vi "Configure PA UTSIGNAL.vi"(8 "error in (no error)":errorcluster, 9 "OFF/ON":u8 max=1 step=1, 10 "Step":T1=1 min=1 max=99 step=1, 11 "VISA resource in":refnum<visa-resource-name>) -> (0 "error out":errorcluster, 3 "VISA resource out":refnum<visa-resource-name>)   [LabVIEW 2025, in "Chroma 19052.lvlib"]
uses:
  <instrlib>/Chroma 19052/Chroma 19052.lvlib
  <instrlib>/Chroma 19052/Public/Utility/Type Def/steps--numeric.ctl
panel:
  # "Set UT SIGNAL on/off"
  # "0 = OFF\n1 = ON"
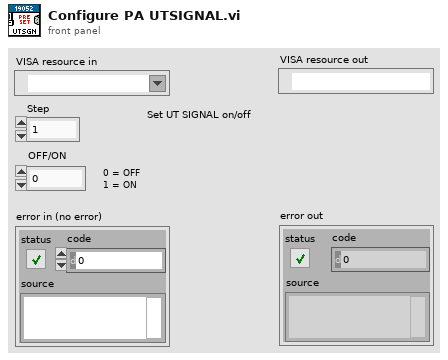
[diagram p1: front panel]
types:
  T1 = typedef "Chroma 19052.lvlib/steps--numeric.ctl" = u8
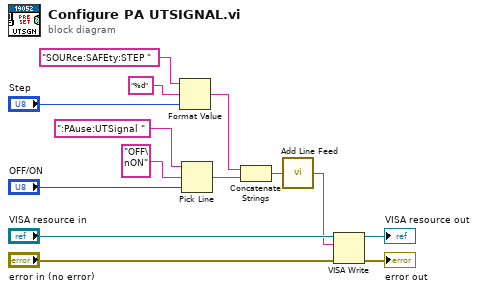
[diagram p0: block diagram]
diagram:
  n1 = Format Value(string ("")="SOURce:SAFEty:STEP ", format string="%d", value (0)="Step") -> (output string=w4:string)
  n2 = Pick Line(string ("")=":PAuse:UTSignal ", multi-line string="OFF\nON", line index="OFF/ON") -> (output string=w5:string)
  n3 = Concatenate Strings(w4, w5) -> (w3:string)
  n4 = call <instrlib>:"Add Line Feed.vi"("Command string"=w3) -> ("Concatenated string"=w2:string)  [unwired: 4 in]
  n5 = VISA Write(VISA resource name="VISA resource in", write buffer=w2, error in (no error)="error in (no error)") -> (VISA resource name out=→"VISA resource out":refnum<visa-resource-name>, error out=→"error out":errorcluster)  [unwired: 1 out]
